vi "PH_SHS_Analysis_Statistician.i attribute.vi"(0 "VI Refnum":refnum<vi>, 2 "CLASS.i attribute":T1={"GUI Refs "={"Status"=refnum, "Result Graph"=refnum, "Mean Data 1"=refnum, "Std Dev Data 1"=refnum, "Mean Data 2"=refnum, "Std Dev Data 2"=refnum, "Mean Data 3"=refnum, "Std Dev Data 3"=refnum, "Dummy Mean"=refnum, "Dummy Std Dev"=refnum, "Export Data"=refnum, "Data 1"=refnum, "Data 2"=refnum, "Data 3"=refnum, "Stat or Trend"=refnum, "Delete"=refnum, "Analyzer"=refnum, "Current Zernike Coefficients"=refnum, "PtV [Lambda]"=refnum, "sample length"=refnum}, "Analyzer"="", "Stat or Trend"=FALSE, "Data 1"=0, "Data 2"=0, "Data 3"=0, "Data"=[], "sample length"=1, "Datasets strored"=0, "Dataarray Size"=0} {"Data"."State" items=["no info", "off/false/out", "on/true/in", "Failure", "Alarm", "Status 1", "Status 2", "Status 3"]; "Data"."Zernicke Coefficients"."2nd Spherical" scale=-2.0..2.0 scale format="%.2f"; "Data"."Zernicke Coefficients"."2nd Coma y" scale=-2.0..2.0 scale format="%.2f"; "Data"."Zernicke Coefficients"."2nd Coma x" scale=-2.0..2.0 scale format="%.2f"; "Data"."Zernicke Coefficients"."2nd Astig 45°" scale=-2.0..2.0 scale format="%.2f"; "Data"."Zernicke Coefficients"."2nd Astig 0°" scale=-2.0..2.0 scale format="%.2f"; "Data"."Zernicke Coefficients"."Trefoil 30°" scale=-2.0..2.0 scale format="%.2f"; "Data"."Zernicke Coefficients"."Trefoil 0°" scale=-2.0..2.0 scale format="%.2f"; "Data"."Zernicke Coefficients"."Spherical" scale=-2.0..2.0 scale format="%.2f"; "Data"."Zernicke Coefficients"."Coma y" scale=-2.0..2.0 scale format="%.2f"; "Data"."Zernicke Coefficients"."Coma x" scale=-2.0..2.0 scale format="%.2f"; "Data"."Zernicke Coefficients"."Astig 45°" scale=-2.0..2.0 scale format="%.2f"; "Data"."Zernicke Coefficients"."Astig 0°" scale=-2.0..2.0 scale format="%.2f"; "Data"."Zernicke Coefficients"."Defocus" scale=-2.0..2.0 scale format="%.2f"; "Data"."Zernicke Coefficients"."Tilt y" scale=-2.0..2.0 scale format="%.2f"; "Data"."Zernicke Coefficients"."Tilt x" scale=-2.0..2.0 scale format="%.2f"}, 3 "Action":T5(ring), 5 "error in (no error)":errorcluster) -> (14 "VI Refnum out":refnum<vi>, 16 "CLASS.i attribute out":T1={"GUI Refs "={"Status"=refnum, "Result Graph"=refnum, "Mean Data 1"=refnum, "Std Dev Data 1"=refnum, "Mean Data 2"=refnum, "Std Dev Data 2"=refnum, "Mean Data 3"=refnum, "Std Dev Data 3"=refnum, "Dummy Mean"=refnum, "Dummy Std Dev"=refnum, "Export Data"=refnum, "Data 1"=refnum, "Data 2"=refnum, "Data 3"=refnum, "Stat or Trend"=refnum, "Delete"=refnum, "Analyzer"=refnum, "Current Zernike Coefficients"=refnum, "PtV [Lambda]"=refnum, "sample length"=refnum}, "Analyzer"="", "Stat or Trend"=FALSE, "Data 1"=0, "Data 2"=0, "Data 3"=0, "Data"=[], "sample length"=1, "Datasets strored"=0, "Dataarray Size"=0} {"Data"."State" items=["no info", "off/false/out", "on/true/in", "Failure", "Alarm", "Status 1", "Status 2", "Status 3"]; "Data"."Zernicke Coefficients"."2nd Spherical" scale=-2.0..2.0 scale format="%.2f"; "Data"."Zernicke Coefficients"."2nd Coma y" scale=-2.0..2.0 scale format="%.2f"; "Data"."Zernicke Coefficients"."2nd Coma x" scale=-2.0..2.0 scale format="%.2f"; "Data"."Zernicke Coefficients"."2nd Astig 45°" scale=-2.0..2.0 scale format="%.2f"; "Data"."Zernicke Coefficients"."2nd Astig 0°" scale=-2.0..2.0 scale format="%.2f"; "Data"."Zernicke Coefficients"."Trefoil 30°" scale=-2.0..2.0 scale format="%.2f"; "Data"."Zernicke Coefficients"."Trefoil 0°" scale=-2.0..2.0 scale format="%.2f"; "Data"."Zernicke Coefficients"."Spherical" scale=-2.0..2.0 scale format="%.2f"; "Data"."Zernicke Coefficients"."Coma y" scale=-2.0..2.0 scale format="%.2f"; "Data"."Zernicke Coefficients"."Coma x" scale=-2.0..2.0 scale format="%.2f"; "Data"."Zernicke Coefficients"."Astig 45°" scale=-2.0..2.0 scale format="%.2f"; "Data"."Zernicke Coefficients"."Astig 0°" scale=-2.0..2.0 scale format="%.2f"; "Data"."Zernicke Coefficients"."Defocus" scale=-2.0..2.0 scale format="%.2f"; "Data"."Zernicke Coefficients"."Tilt y" scale=-2.0..2.0 scale format="%.2f"; "Data"."Zernicke Coefficients"."Tilt x" scale=-2.0..2.0 scale format="%.2f"}, 19 "error out":errorcluster)   [LabVIEW 2014, in "PH_SHS_Analysis_Statistician.lvlib"]
doc: "This is a so-called functional global variable. It manages the access to a global variable in a thread-safe way. \n\nHere the attribute data of all instances of THIS class are stored. This is done for performance reasons.\n\nLicense Agreement for this software:\n\nCopyright (C)\nGesellschaft für Schwerionenforschung, GSI\nPlanckstr. 1\n64291 Darmstadt\nGermany\n\nContact: D.Beck@gsi.de \n\nThis program is free software; you can redistribute it and/or modify it under the terms of the GNU General Public License as published by the Free Software Foundation; either version 2 of the license, or (at your option) any later version.\n\nThis program is distributed in the hope that it will be useful, but WITHOUT ANY WARRANTY; without even the implied warranty of MERCHANTABILITY or FITNESS FOR A PARTICULAR PURPOSE. See the GNU General License for more details (http://www.gnu.org).\n\nGesellschaft für Schwerionenforschung, GSI\nPlanckstr. 1, 64291 Darmstadt, Germany\nFor all questions and ideas contact: M.Richter@gsi.de, H.Brand@gsi.de or D.Beck@gsi.de.\nLast update: 17-JUN-2004"
uses:
  PH_SHS_Analysis_Statistician.lvlib
  PH_SHS_Analysis_Statistician.i attribute.ctl
  PH_SHS_Analysis/PH_SHS_Analysis.Zernike Dataset.ctl
  PH_Basics/PH_StatusHandler/PH_StatusHandler.Status.ctl
  PH_SHS_Analysis/PH_SHS_Analysis.Zernike Coefficients.ctl
  CS_Core/CSSystem/CoreDefs/CoreDefs.error_type.ctl
  CS_Core/CSSystem/CoreLib/CoreLib.lvlib
  PH_SHS_Analysis/PH_SHS_Analysis.lvlib
  PH_Basics/PH_StatusHandler/PH_StatusHandler.lvlib
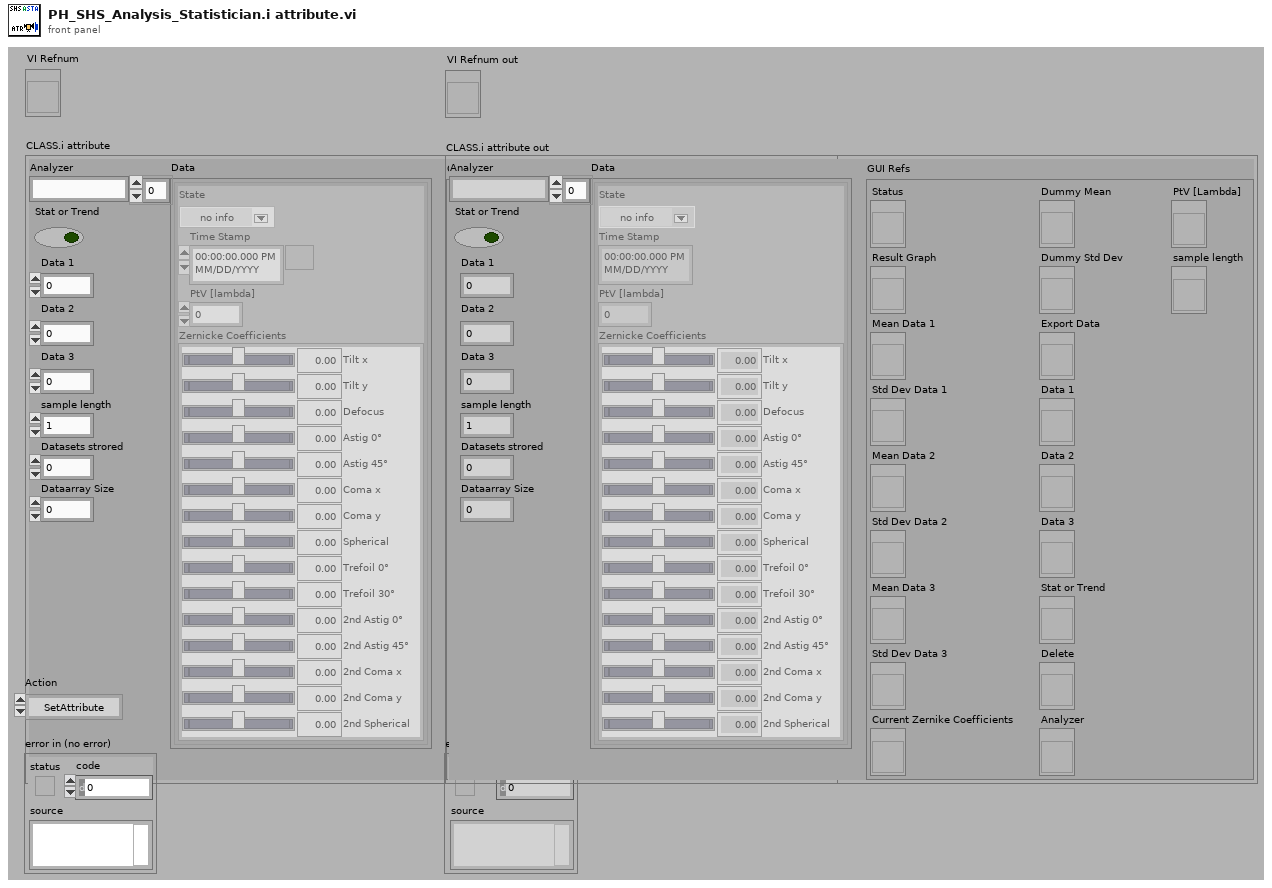
[diagram p1: front panel]
types:
  T1 = typedef "PH_SHS_Analysis_Statistician.lvlib/PH_SHS_Analysis_Statistician.i attribute.ctl" = cluster{"GUI Refs ":cluster{"Status":refnum<vi>, "Result Graph":refnum<vi>, "Mean Data 1":refnum<vi>, "Std Dev Data 1":refnum<vi>, "Mean Data 2":refnum<vi>, "Std Dev Data 2":refnum<vi>, "Mean Data 3":refnum<vi>, "Std Dev Data 3":refnum<vi>, "Dummy Mean":refnum<vi>, "Dummy Std Dev":refnum<vi>, "Export Data":refnum<vi>, "Data 1":refnum<vi>, "Data 2":refnum<vi>, "Data 3":refnum<vi>, "Stat or Trend":refnum<vi>, "Delete":refnum<vi>, "Analyzer":refnum<vi>, "Current Zernike Coefficients":refnum<vi>, "PtV [Lambda]":refnum<vi>, "sample length":refnum<vi>}, "Analyzer":string, "Stat or Trend":bool, "Data 1":i16, "Data 2":i16, "Data 3":i16, "Data":T2[], "sample length":i32, "Datasets strored":i32, "Dataarray Size":i32}
  T2 = typedef "PH_SHS_Analysis.lvlib/PH_SHS_Analysis.Zernike Dataset.ctl" = cluster{"State":T3, "Time Stamp":timestamp, "PtV [lambda]":dbl, "Zernicke Coefficients":T4}
  T3 = typedef "PH_StatusHandler.lvlib/PH_StatusHandler.Status.ctl" = i16
  T4 = typedef "PH_SHS_Analysis.lvlib/PH_SHS_Analysis.Zernike Coefficients.ctl" = cluster{"Tilt x":dbl, "Tilt y":dbl, "Defocus":dbl, "Astig 0°":dbl, "Astig 45°":dbl, "Coma x":dbl, "Coma y":dbl, "Spherical":dbl, "Trefoil 0°":dbl, "Trefoil 30°":dbl, "2nd Astig 0°":dbl, "2nd Astig 45°":dbl, "2nd Coma x":dbl, "2nd Coma y":dbl, "2nd Spherical":dbl}
  T5 = enum16{"SetAttribute", "GetAttribute", "CreateAttribute", "DestroyAttribute", "DestroyAllAtributes"}
  T6 = typedef "CoreDefs.error_type.ctl" = enum16{"no error", "can't load process", "can't unload process", "process does not exist", "can't install process", "can't remove process", "unknown function", "time out", "can't execute function", "duplicate queue name", "super not found", "caller queue invalid", "can't ping process", "unknown error", "VISA Error", "VISA timeout", "GPIB timeout", "GPIB error", "communication error", "data type mismatch", "can't read data from OPC server", "can't write data to OPC server", "OET error", "function not implemented", "process already exists", "invalid Shared Variable name", "error writing Shared Variable", "error reading Shared Variable", "invalid client name", "corrupt database", "unknown class", "call not authorized", "parameter out of range", "OET timeout: can't get data to modify", "invalid queue name", "requested operation incompatible with current state", "event undefined", "event disabled", "state undefined", "caller is not a friend", "EventBuilder: bad eventID", "EventBuilder: no DAQ devices", "a thread must not stop itself", "UNUSED ELEMENT4", "DiscArchiver: eventData incomplete", "DiscArchiver: eventData does not belong to run", "DiscArchiver: can't open file", "DiscArchiver: can't write to file", "DiscArchiver: available disc space low", "can't acquire semaphore", "error reading data from database", "notifier object is not existing", "can't register process", "can't unregister process", "illegal event type", "object disabled", "object already exists", "can't change state", "Instrument not found", "no connection to remote node", "invalid reference", "N/A", "UNUSED ELEMENT 1", "element not found", "illegal TCP/IP connection detected", "object does not exist", "invalid access ID", "unknown CS system", "invalid privilige", "unsupported data type", "unsupported server type", "IO server already exists", "Shared Variable already exists"}
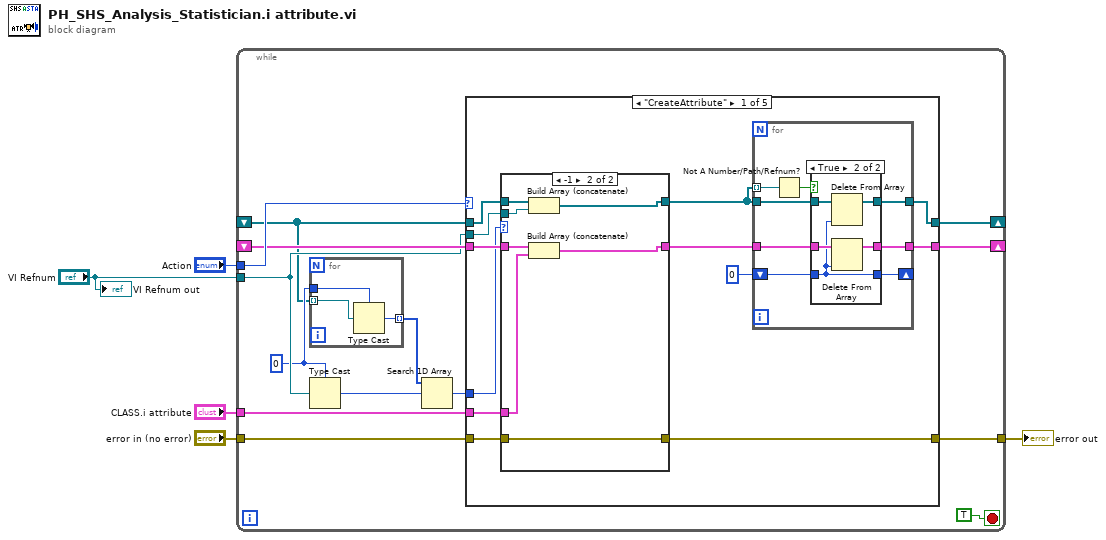
[diagram p0: block diagram]
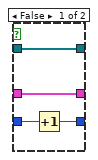
[diagram p2: hidden frame]
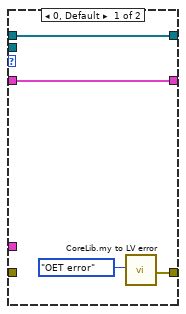
[diagram p3: hidden frame]
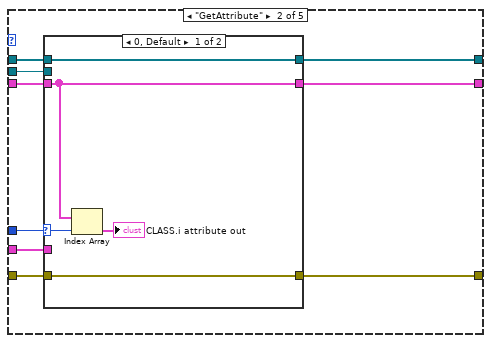
[diagram p4: hidden frame]
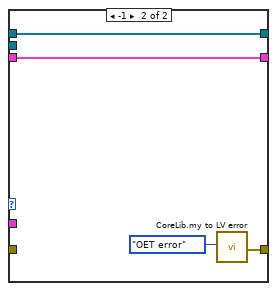
[diagram p5: hidden frame]
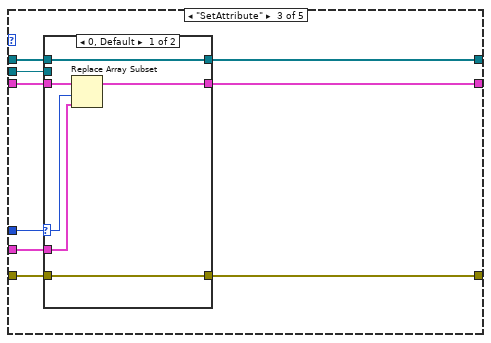
[diagram p6: hidden frame]
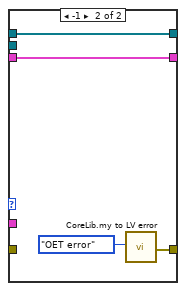
[diagram p7: hidden frame]
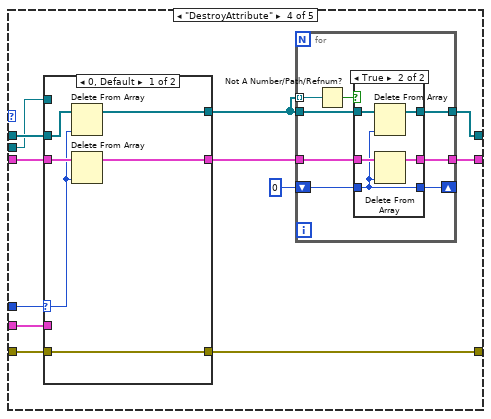
[diagram p8: hidden frame]
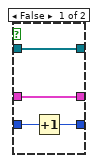
[diagram p9: hidden frame]
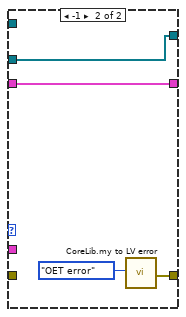
[diagram p10: hidden frame]
diagram:
  n1 = while {
    shift-right: [w13] -> _
    shift-left: _ -> [w14]
    tunnel: "Action" -> [w18]
    shift-right: [w15] -> _
    shift-left: _ -> [w6]
    tunnel: "error in (no error)" -> [w17]
    tunnel: [w16] -> w3
    tunnel: "CLASS.i attribute" -> [w12]
    tunnel: "VI Refnum" -> [w9]
    stop <- TRUE stop-if-true
    w8 = 0
    n2 = for {
      tunnel: w8 -> [w22]
      tunnel: [w21] -> w7 mode=indexing
      tunnel: w6 -> [w20] mode=indexing
      n3 = Type Cast(type=w22, x=w20) -> (*(type *) &x=w21:i32)
    }
    n4 = Type Cast(type=w8, x=w9) -> (*(type *) &x=w10:i32)
    n5 = Search 1D Array(1D array=w7, element=w10) -> (index of element=w11:i32)  [unwired: 1 in]
    n6 = case shown="\"CreateAttribute\"" w18 {
      tunnel: w6 -> [w32 w69 w87 w109 _]
      tunnel: w9 -> [w31 w67 w85 w108 _]
      tunnel: w17 -> [w34 w71 w89 w111 w139]
      tunnel: [w33 w70 w88 w110 w139] -> w16
      tunnel: [w26 w68 w86 w103 _] -> w15
      tunnel: w14 -> [w30 w66 w84 w107 _]
      tunnel: [w25 w65 w83 w101 _] -> w13
      tunnel: w12 -> [w29 w64 w82 w106 _]
      tunnel: w11 -> [w28 w63 w81 w105 _]
      frame "CreateAttribute" {
        n7 = case shown="-1" w28 {
          tunnel: w34 -> [_ w62]
          tunnel: [w54 w62] -> w33
          tunnel: w32 -> [w53 w61]
          tunnel: [w53 w60] -> w24
          tunnel: w31 -> [_ w59]
          tunnel: w30 -> [w52 w58]
          tunnel: [w52 w57] -> w23
          tunnel: w29 -> [_ w56]
          frame 0, Default {
            n8 = call "CoreLib.my to LV error.vi"("ErrorTypes"=CoreDefs.error_type."OET error") -> ("myErrorCluster"=w54:errorcluster)  [unwired: 17 in, 1 out]
          }
          frame -1 {
            n9 = Build Array (concatenate)(w61, w59) -> (w60:refnum<vi>[])
            n10 = Build Array (concatenate)(w58, w56) -> (w57:T1[])
          }
        }
        n11 = for {
          tunnel: w24 -> [w39]
          tunnel: [w38] -> w26
          tunnel: [w42] -> w25
          tunnel: w23 -> [w41]
          tunnel: w24 -> [w37] mode=indexing
          shift-right: [w36] -> _
          shift-left: 0 -> [w35]
          n12 = Not A Number/Path/Refnum?(number/path/refnum=w37) -> (NaN/Path/Refnum?=w40:bool)
          n13 = case shown="True" w40 {
            tunnel: [w46 w51] -> w42
            tunnel: w41 -> [w46 w50]
            tunnel: [w45 w48] -> w38
            tunnel: w39 -> [w45 w49]
            tunnel: w35 -> [w44 w47]
            tunnel: [w43 w47] -> w36
            frame False {
              n14 = Increment(x=w44) -> (x+1=w43:i32)
            }
            frame True {
              n15 = Delete From Array(array=w49, index=w47) -> (array with subset deleted=w48:refnum<vi>[])  [unwired: 1 in, 1 out]
              n16 = Delete From Array(array=w50, index=w47) -> (array with subset deleted=w51:T1[])  [unwired: 1 in, 1 out]
            }
          }
        }
      }
      frame "GetAttribute" {
        n17 = case shown="0, Default" w63 {
          selector: w63 -> [w74 _]
          tunnel: w71 -> [w76 _]
          tunnel: [w76 w79] -> w70
          tunnel: w69 -> [w75 w78]
          tunnel: [w75 w78] -> w68
          tunnel: w67 -> [_ _]
          tunnel: w66 -> [w73 w77]
          tunnel: [w73 w77] -> w65
          tunnel: w64 -> [_ _]
          frame 0, Default {
            n18 = Index Array(array=w73, index=w74) -> (element=→"CLASS.i attribute out":T1)
          }
          frame -1 {
            n19 = call "CoreLib.my to LV error.vi"("ErrorTypes"=CoreDefs.error_type."OET error") -> ("myErrorCluster"=w79:errorcluster)  [unwired: 17 in, 1 out]
          }
        }
      }
      frame "SetAttribute" {
        n20 = case shown="0, Default" w81 {
          selector: w81 -> [w91 _]
          tunnel: w89 -> [w95 _]
          tunnel: [w95 w98] -> w88
          tunnel: w87 -> [w94 w97]
          tunnel: [w94 w97] -> w86
          tunnel: w85 -> [_ _]
          tunnel: w84 -> [w93 w96]
          tunnel: [w92 w96] -> w83
          tunnel: w82 -> [w90 _]
          frame 0, Default {
            n21 = Replace Array Subset(array=w93, new element=w90, index=w91) -> (w92:T1[])
          }
          frame -1 {
            n22 = call "CoreLib.my to LV error.vi"("ErrorTypes"=CoreDefs.error_type."OET error") -> ("myErrorCluster"=w98:errorcluster)  [unwired: 17 in, 1 out]
          }
        }
      }
      frame "DestroyAttribute" {
        n23 = case shown="0, Default" w105 {
          selector: w105 -> [w130 _]
          tunnel: w111 -> [w134 _]
          tunnel: [w134 w137] -> w110
          tunnel: w109 -> [w133 w136]
          tunnel: [w132 w136] -> w102
          tunnel: w108 -> [_ _]
          tunnel: w107 -> [w131 w135]
          tunnel: [w129 w135] -> w100
          tunnel: w106 -> [_ _]
          frame 0, Default {
            n24 = Delete From Array(array=w133, index=w130) -> (array with subset deleted=w132:refnum<vi>[])  [unwired: 1 in, 1 out]
            n25 = Delete From Array(array=w131, index=w130) -> (array with subset deleted=w129:T1[])  [unwired: 1 in, 1 out]
          }
          frame -1 {
            n26 = call "CoreLib.my to LV error.vi"("ErrorTypes"=CoreDefs.error_type."OET error") -> ("myErrorCluster"=w137:errorcluster)  [unwired: 17 in, 1 out]
          }
        }
        n27 = for {
          tunnel: w102 -> [w116]
          tunnel: [w115] -> w103
          tunnel: [w119] -> w101
          tunnel: w100 -> [w118]
          tunnel: w102 -> [w114] mode=indexing
          shift-right: [w113] -> _
          shift-left: 0 -> [w112]
          n28 = Not A Number/Path/Refnum?(number/path/refnum=w114) -> (NaN/Path/Refnum?=w117:bool)
          n29 = case shown="True" w117 {
            tunnel: [w123 w128] -> w119
            tunnel: w118 -> [w123 w127]
            tunnel: [w122 w125] -> w115
            tunnel: w116 -> [w122 w126]
            tunnel: w112 -> [w121 w124]
            tunnel: [w120 w124] -> w113
            frame False {
              n30 = Increment(x=w121) -> (x+1=w120:i32)
            }
            frame True {
              n31 = Delete From Array(array=w126, index=w124) -> (array with subset deleted=w125:refnum<vi>[])  [unwired: 1 in, 1 out]
              n32 = Delete From Array(array=w127, index=w124) -> (array with subset deleted=w128:T1[])  [unwired: 1 in, 1 out]
            }
          }
        }
      }
      frame "DestroyAllAtributes" {
      }
    }
  }
  "error out" <- w3
  "VI Refnum out" <- "VI Refnum"
